vi "Log Event.vi"(1 "Event Description":string) -> ()   [LabVIEW 2012]
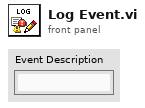
[diagram p1: front panel]
types:
  T1 = enum16{"open", "replace", "create", "open or create", "replace or create", "replace or create with confirmation"}
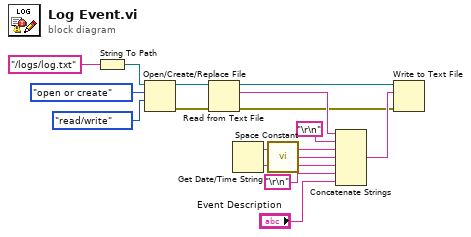
[diagram p0: block diagram]
diagram:
  n1 = String To Path(string="/logs/log.txt") -> (path=w16:path)
  n2 = Open/Create/Replace File(file path (use dialog)=w16, operation (0:open)=T1."open or create", access (0:read/write)=enum16{"read/write", "read-only", "write-only"}."read/write") -> (refnum out=w12:refnum<file>, error out=w11:errorcluster)  [unwired: 3 in, 1 out]
  n3 = Read from Text File(file (use dialog)=w12, error in=w11) -> (refnum out=w2:refnum<file>, text=w10:string, error out=w1:errorcluster)  [unwired: 2 in, 1 out]
  n4 = Get Date/Time String() -> (date string=w8:string, time string=w6:string)  [unwired: 3 in]
  n5 = call <vilib>:"Space Constant.vi"() -> ("String"=w7:string)
  n6 = Concatenate Strings(w10, "\r\n", w8, w7, w6, "\r\n", "Event Description") -> (w3:string)
  n7 = Write to Text File(file (use dialog)=w2, text=w3, error in=w1) -> ()  [unwired: 1 in, 3 out]
